vi "写标定功率检测值解析.vi"(9 "读取的字节":i32, 10 "响应":string) -> ()   [LabVIEW 2015]
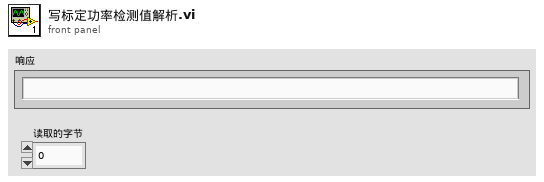
[diagram p1: front panel]
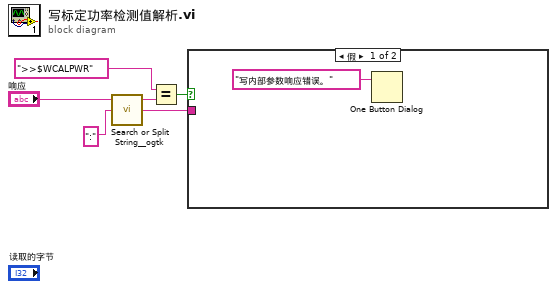
[diagram p0: block diagram]
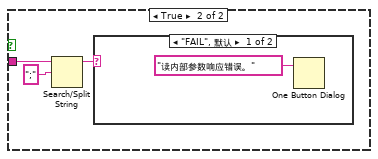
[diagram p2: hidden frame]
diagram:
  n1 = call <userlib>:"Search or Split String__ogtk.vi"("search string/char (-)"=":", "string"="响应") -> ("substring after match"=w1:string, "substring before match"=w4:string)  [unwired: 1 in, 1 out]
  n2 = Equal?(x=">>$WCALPWR" ("search string/char (-)"), y=w4) -> (x = y?=w2:bool)
  n3 = case shown="假" w2 {
    tunnel: w1 -> [_ w9]
    frame False {
      n4 = One Button Dialog(message="写内部参数响应错误。" ("消息")) -> ()  [unwired: 1 in, 1 out]
    }
    frame True {
      n5 = Search/Split String(string=w9, search string/char (-)=";" ("搜索字符串/字符(-)")) -> (substring before match=w8:string)  [unwired: 1 in, 2 out]
      n6 = case shown="\"FAIL\", 默认" w8 {
        frame "FAIL", Default {
          n7 = One Button Dialog(message="读内部参数响应错误。" ("消息")) -> ()  [unwired: 1 in, 1 out]
        }
        frame "OK" {
        }
      }
    }
  }
